vi "Read Text File.vi"() -> ()   [LabVIEW 2022 SP3]
panel:
  out "sum":i16
  in  "String":string
  out "length":i32
  out "error out":errorcluster
  out "text":string
  in  "file path (use dialog)":path
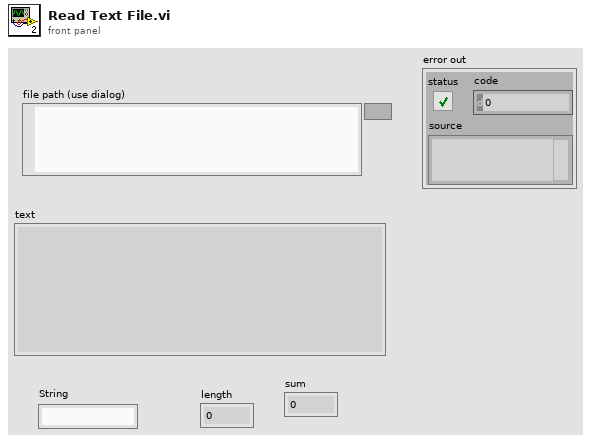
[diagram p1: front panel]
types:
  T1 = enum16{"open", "replace", "create", "open or create", "replace or create", "replace or create with confirmation"}
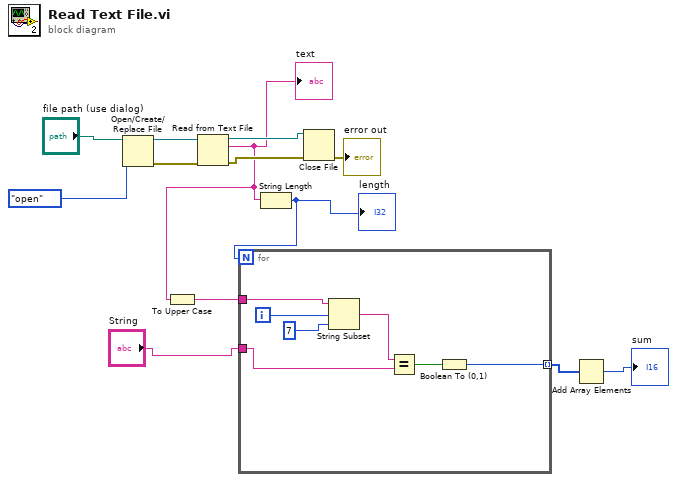
[diagram p0: block diagram]
diagram:
  n1 = Open/Create/Replace File(file path (use dialog)="file path (use dialog)", operation (0:open)=T1."open") -> (refnum out=w11:refnum<file>, error out=w10:errorcluster)  [unwired: 4 in, 1 out]
  n2 = Read from Text File(file (use dialog)=w11, error in=w10) -> (refnum out=w9:refnum<file>, text=w5:string, error out=w8:errorcluster)  [unwired: 2 in, 1 out]
  "text" <- w5
  n3 = To Upper Case(1:w5) -> (0:w4:string)
  n4 = String Length(string=w5) -> (length=w6:i32)
  "length" <- w6
  n5 = for {
    N: w6 -> [_]
    tunnel: w4 -> [w20]
    tunnel: "String" -> [w16]
    tunnel: [w14] -> w2 mode=indexing
    i -> [w19]
    n6 = String Subset(string=w20, offset (0)=w19, length (rest)=7 ("length (rest)")) -> (substring=w17:string)
    n7 = Equal?(x=w17, y=w16) -> (x = y?=w15:bool)
    n8 = Boolean To (0,1)(Boolean=w15) -> (0, 1=w14:i16)
  }
  n9 = Close File(refnum=w9, error in=w8) -> (error out=→"error out":errorcluster)  [unwired: 1 out]
  n10 = Add Array Elements(numeric array=w2) -> (sum=→"sum":i16)
